vi "Turnrate_to_Side_Drag.vi"(1 "Turn Rate":dbl) -> (0 "Side Drag":dbl)   [LabVIEW 2009]
uses:
  <vilib>/gmath/NI_Gmath.lvlib
panel:
  in  "Drag / Turn Rate":cluster{"F":dbl, "V":dbl}[](array[cluster])=[{"F"=-4.18, "V"=-120.54}, {"F"=-3.93, "V"=-119.78}, {"F"=-2.55, "V"=-100.62}, {"F"=-1.33, "V"=-76.36}, {"F"=-0.38, "V"=-40.02}, {"F"=0.0, "V"=0.0}, {"F"=0.38, "V"=38.01}, {"F"=1.34, "V"=73.52}, {"F"=2.52, "V"=99.54}, {"F"=3.88, "V"=118.38}, {"F"=3.98, "V"=119.78}]
  # "Drag is in N\nTurn Rate in deg/s"
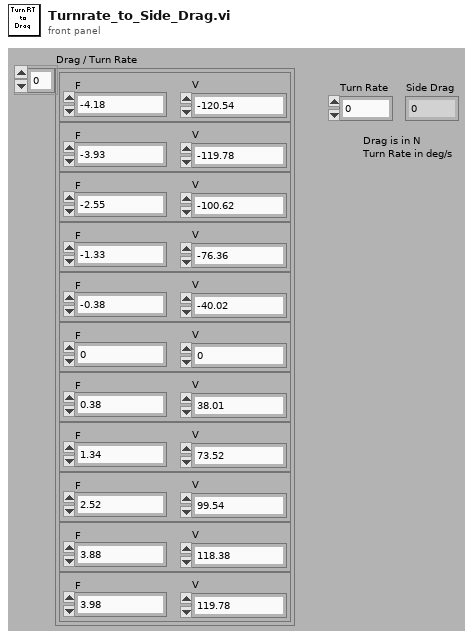
[diagram p1: front panel]
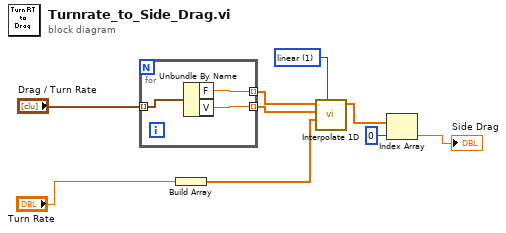
[diagram p0: block diagram]
diagram:
  w9 = 1 items=["nearest", "linear", "spline", "cubic Hermite", "Lagrange"] ("method")
  n1 = for {
    tunnel: "Drag / Turn Rate" -> [w12] mode=indexing
    tunnel: [w11] -> w7 mode=indexing
    tunnel: [w10] -> w6 mode=indexing
    n2 = Unbundle By Name(w12) -> ("F"=w11:dbl, "V"=w10:dbl)
  }
  n3 = Build Array("Turn Rate") -> (w1:dbl[])
  n4 = call <vilib>:"Interpolate 1D.vi"("method"=w9, "xi"=w1, "X"=w6, "Y"=w7) -> ("yi"=w4:dbl[])  [unwired: 5 in, 2 out]
  n5 = Index Array(array=w4, index=0) -> (element=→"Side Drag":dbl)
